vi "Channels.Filter.vi"(8 "error in (no error)":errorcluster, 11 "state variables in":T1) -> (0 "error out":errorcluster, 3 "state variables out":T1)   [LabVIEW 2015, in "Stations.Overview.lvlib"]
uses:
  Stations.Overview.lvlib
  Types/Overview.StateVariables.ctl
  Types/Overview.Channels.ctl
  <vilib>/NI Veristand/Execution/Workspace/SystemStateEventRef.ctl
  <vilib>/NI Veristand/Execution/Workspace/Target State Info.ctl
  <vilib>/NI Veristand/Execution/Workspace/Target State.ctl
  <vilib>/NI Veristand/Execution/Workspace/WorkspaceAPI.ctl
  NationalInstruments.VeriStand.ClientAPI
  Execution GUI/Types/Execute.UserEventRefs.ctl
  <vilib>/NI Veristand/Execution/Workspace/SystemStateRegEventRef.ctl
  <vilib>/NI Veristand/Execution/WaveformStreaming/Waveform Data Watcher Event Data (DBL).ctl
  <vilib>/NI Veristand/Execution/WaveformStreaming/WaveformStreamSpecification.ctl
  NationalInstruments.VeriStand
  <vilib>/NI Veristand/Execution/Workspace/NI_VS Workspace ExecutionAPI.lvlib
  Execution GUI/Station.Execution.lvlib
  <vilib>/NI Veristand/Execution/WaveformStreaming/NI_VS Waveform Streaming Interface.lvlib
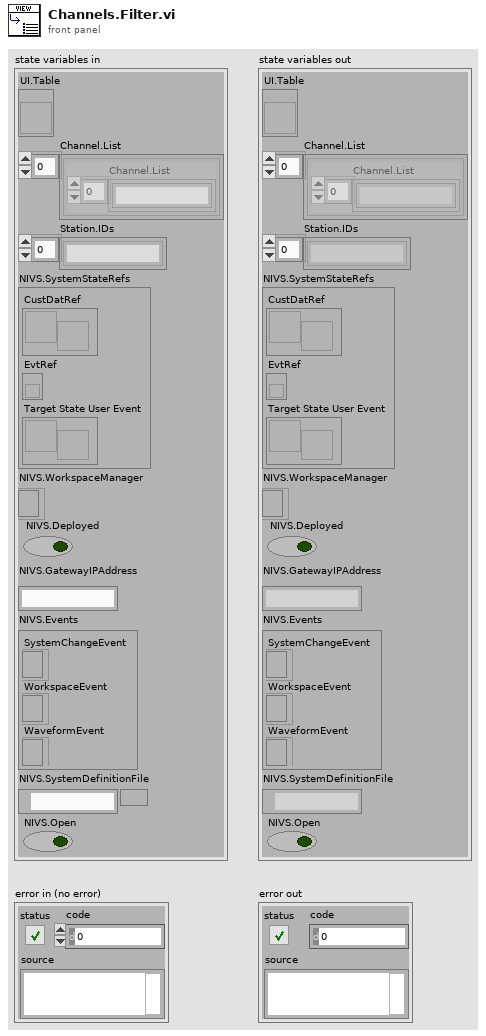
[diagram p1: front panel]
types:
  T1 = typedef "Stations.Overview.lvlib/Overview.StateVariables.ctl" = cluster{"UI.Table":refnum<vi>, "Channel.List":T2[], "Station.IDs":string[], "NIVS.SystemStateRefs":T3, "NIVS.WorkspaceManager":T4, "NIVS.Deployed":bool, "NIVS.GatewayIPAddress":string, "NIVS.Events":T5, "NIVS.SystemDefinitionFile":path, "NIVS.Open":bool}
  T2 = typedef "Stations.Overview.lvlib/Overview.Channels.ctl" = cluster{"Channel.List":string[]}
  T3 = typedef "NI_VS Workspace ExecutionAPI.lvlib/SystemStateEventRef.ctl" = cluster{"CustDatRef":refnum<user-event>, "EvtRef":refnum<k27>, "Target State User Event":refnum<user-event>}
  T4 = typedef "NI_VS Workspace ExecutionAPI.lvlib/WorkspaceAPI.ctl" = refnum<k24>
  T5 = typedef "Station.Execution.lvlib/Execute.UserEventRefs.ctl" = cluster{"SystemChangeEvent":T6, "WorkspaceEvent":refnum<event-registration>, "WaveformEvent":refnum<event-registration>}
  T6 = typedef "NI_VS Workspace ExecutionAPI.lvlib/SystemStateRegEventRef.ctl" = refnum<event-registration>
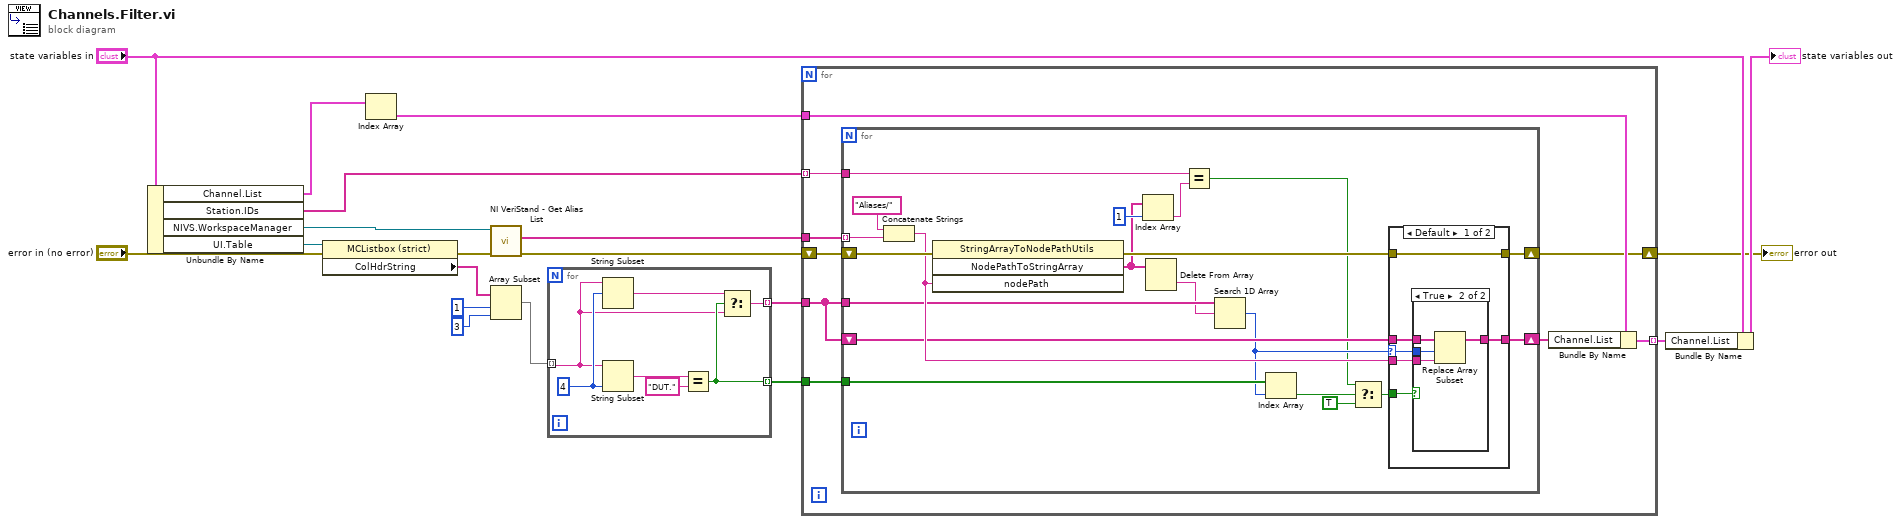
[diagram p0: block diagram]
diagram:
  n1 = Unbundle By Name("state variables in") -> ("Channel.List"=w7:T2[], "Station.IDs"=w17:string[], "NIVS.WorkspaceManager"=w15:T4, "UI.Table"=w14:refnum<vi>)
  n2 = property class="MCListbox (strict)"(reference=w14, error in="error in (no error)") -> (error out=w16:errorcluster, "ColHdrString"=w12:string[])  [unwired: 1 out]
  n3 = Index Array(array=w7) -> (element=w6:T2)  [unwired: 1 in]
  n4 = call <vilib>:"NI VeriStand - Get Alias List.vi"("error in (no error)"=w16, "WorkspaceManager in"=w15) -> ("error out"=w9:errorcluster, "Aliases"=w8:string[])  [unwired: 6 in, 2 out]
  n5 = Array Subset(array=w12, index=1 ("length"), length=3 ("index")) -> (w2:string[])
  n6 = for {
    tunnel: w2 -> [w21] mode=indexing
    tunnel: [w24] -> w3 mode=indexing
    tunnel: [w20] -> w1 mode=indexing
    w23 = 4 ("length (rest)")
    n7 = String Subset(string=w21, offset (0)=w23) -> (substring=w22:string)  [unwired: 1 in]
    n8 = String Subset(string=w21, length (rest)=w23) -> (substring=w26:string)  [unwired: 1 in]
    n9 = Equal?(x=w26, y="DUT.") -> (x = y?=w24:bool)
    n10 = Select(t=w22, s=w24, f=w21) -> (s? t:f=w20:string)
  }
  n11 = for {
    tunnel: w17 -> [w35] mode=indexing
    tunnel: w8 -> [w33]
    tunnel: w1 -> [w32]
    tunnel: w6 -> [w31]
    tunnel: [w29] -> w4 mode=indexing
    shift-right: [w28] -> w5
    shift-left: w9 -> [w34]
    tunnel: w3 -> [w27]
    n12 = for {
      tunnel: w35 -> [w50]
      shift-right: [w43] -> w28
      shift-left: w34 -> [w53]
      tunnel: w33 -> [w54] mode=indexing
      tunnel: w32 -> [w46]
      shift-right: [w44] -> w30
      shift-left: w32 -> [w45]
      tunnel: w27 -> [w41]
      n13 = Concatenate Strings("Aliases/" ("string"), w54) -> (w48:string)
      n14 = invoke class="StringArrayToNodePathUtils" method="NodePathToStringArray"(error in=w53, "nodePath"=w48) -> (error out=w49:errorcluster, "NodePathToStringArray"=w47:string[])  [unwired: 2 in, 2 out]
      n15 = Index Array(array=w47, index=1) -> (element=w51:string)
      n16 = Delete From Array(array=w47) -> (deleted portion=w42:string)  [unwired: 2 in, 1 out]
      n17 = Equal?(x=w50, y=w51) -> (x = y?=w39:bool)
      n18 = Search 1D Array(1D array=w46, element=w42) -> (index of element=w40:i32)  [unwired: 1 in]
      n19 = Index Array(array=w41, index=w40) -> (element=w37:bool)
      n20 = Select(t=w39, s=w37, f=TRUE) -> (s? t:f=w36:bool)
      n21 = case shown="Default" w40 {
        selector: w40 -> [w60 _]
        tunnel: w45 -> [w61 w68]
        tunnel: w48 -> [w59 _]
        tunnel: [w58 w68] -> w44
        tunnel: [w57 w67] -> w43
        tunnel: w49 -> [w57 w67]
        tunnel: w36 -> [w56 _]
        frame Default {
          n22 = case shown="True" w56 {
            tunnel: w61 -> [w62 w66]
            tunnel: w60 -> [_ w65]
            tunnel: w59 -> [_ w64]
            tunnel: [w62 w63] -> w58
            frame False {
            }
            frame True {
              n23 = Replace Array Subset(array=w66, new element=w64, index=w65) -> (w63:string[])
            }
          }
        }
        frame -1 {
        }
      }
    }
    n24 = Bundle By Name(cluster=w31, "Channel.List"=w30) -> (w29:T2)
  }
  "error out" <- w5
  n25 = Bundle By Name(cluster="state variables in", "Channel.List"=w4) -> (→"state variables out":T1)
